vi "Write Artist.vi"(8 "error in (no error)":errorcluster, 10 "Artist":string, 11 "Song in":refnum<class "Song.lvclass">) -> (0 "error out":errorcluster, 3 "Song out":refnum<class "Song.lvclass">)   [LabVIEW 2015, in "Song.lvclass"]
uses:
  Song.lvclass
  Song.lvclass/Song.ctl
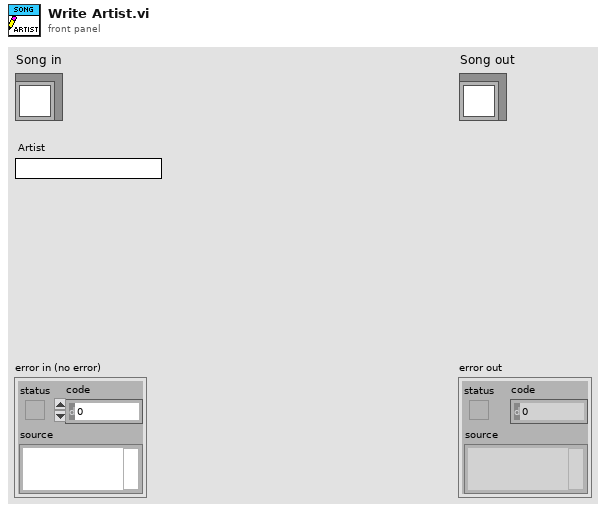
[diagram p1: front panel]
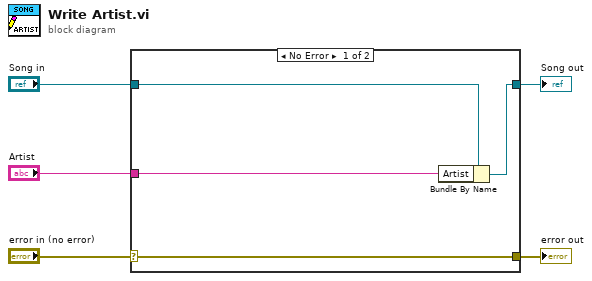
[diagram p0: block diagram]
diagram:
  n1 = case shown="No Error" "error in (no error)" {
    selector: "error in (no error)" -> [w9 w10]
    tunnel: [w9 w10] -> w4
    tunnel: [w7 w11] -> w2
    tunnel: "Song in" -> [w8 w11]
    tunnel: "Artist" -> [w6 _]
    frame No Error {
      n2 = Bundle By Name(cluster=w8, "Artist"=w6) -> (w7:refnum<class "Song.lvclass">)
    }
    frame Error {
    }
  }
  "error out" <- w4
  "Song out" <- w2
